vi "host.vi"() -> ()   [LabVIEW 2020]
uses:
  <vilib>/Analysis/baseanly.llb/Real A x B.vi
  <vilib>/Analysis/7linalg.llb/Real Cholesky Factorization.vi
  <vilib>/Analysis/7linalg.llb/Real Transpose Matrix.vi
  <vilib>/Analysis/baseanly.llb/Full Cholesky Factorization.vi
  <vilib>/Analysis/baseanly.llb/Full Real Matrix Cholesky Factorization.vi
  <vilib>/Analysis/baseanly.llb/Real Inverse Matrix.vi
  <vilib>/Analysis/Matrix/Numeric/Conversions/Matrix To Array - RM.vi
  <vilib>/FPGAPlugInAG/cRIO-9035/niLvFpga_Open_cRIO-9035.vi
  <vilib>/rvi/interface/common/dynamic/niFpgaDynamicAddResources.vi
  <vilib>/Utility/error.llb/Error Cluster From Error Code.vi
  <vilib>/rvi/errors/niLvFpgaAdjustHostInterfaceError.vi
  <vilib>/FPGAPlugInAG/Dynamic/niLvFpga_Run_Dynamic.vi
  <vilib>/FPGAPlugInAG/Dynamic/niLvFpga_Close_Dynamic.vi
  <vilib>/rvi/interface/nirviOpenFPGA/nirviOpenFPGA.xnode
  FPGA Bitfiles/labviewfpgacheck_FPGATarget_target_WT8zXaMNSug.lvbitx
  target.vi
  <vilib>/rvi/interface/nirviMethod/nirviMethod.xnode
  <vilib>/rvi/interface/nirviCloseFPGA/nirviCloseFPGA.xnode
  <vilib>/FPGAPlugInAG/Dynamic/niLvFpga_WriteFifo_Dynamic.vi
  <vilib>/rvi/errors/niLvFpgaMergeErrorWithErrorCode.vi
  <vilib>/FPGAPlugInAG/Dynamic/niLvFpga_ReadFifo_Dynamic.vi
  <vilib>/Analysis/NI_AALBase.lvlib
  <vilib>/Analysis/NI_AALPro.lvlib
  <vilib>/Analysis/Matrix/NI_Matrix.lvlib
panel:
  out "B - LabVIEW code":dbl[][](array[numeric])
  out "sum of error":dbl
  out "B - FPGA code":sgl[][](array[numeric])
  out "A":sgl[][](array[numeric])
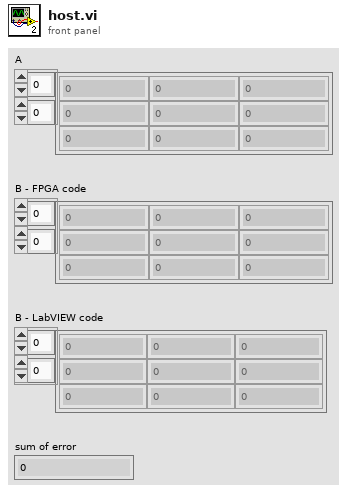
[diagram p1: front panel]
types:
  T1 = typedef "NI_Matrix.lvlib/RealMatrix.ctl" = dbl[][]
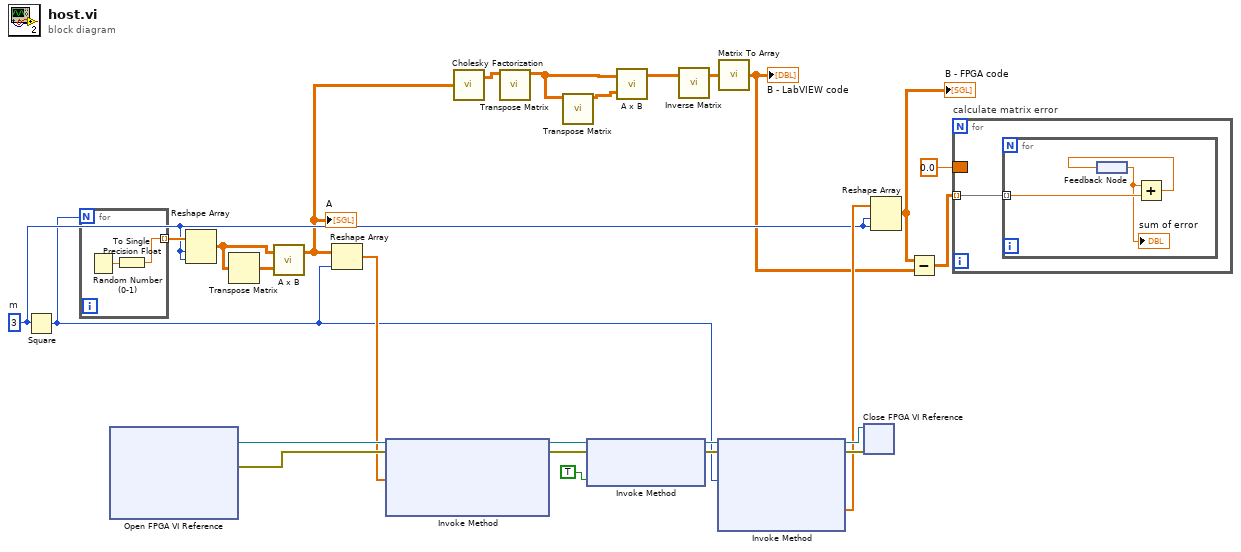
[diagram p0: block diagram]
diagram:
  w10 = 3  # m
  n1 = Square(x=w10) -> (x^2=w9:i32)
  n2 = for {
    N: w9 -> [_]
    tunnel: [w27] -> w13 mode=indexing
    n3 = Random Number (0-1)() -> (number: 0 to 1=w28:dbl)
    n4 = To Single Precision Float(number=w28) -> (single precision float=w27:sgl)
  }
  n5 = xnode "Open FPGA VI Reference"() -> ("FPGA VI Reference Out"=w25:refnum<k20>, "error out"=w24:errorcluster)  [unwired: 2 in]
  n6 = Reshape Array(w13, w10, w10) -> (w11:sgl[][])
  n7 = Transpose Matrix(1:w11) -> (0:w12:dbl[][])
  n8 = call-poly <vilib>:"A x B.vi"("B"=w12, "A"=w11) -> ("A x B"=w6:T1)  [unwired: 1 out]
  "A" <- w6
  n9 = Reshape Array(w6, w9) -> (w19:dbl[])
  n10 = xnode "Invoke Method"("FPGA VI Reference In"=w25, "error in"=w24, "Data"=w19) -> ("FPGA VI Reference Out"=w15:refnum<k20>, "error out"=w14:errorcluster)  [unwired: 1 in, 1 out]
  n11 = call-poly <vilib>:"Cholesky Factorization.vi"("A"=w6) -> ("Cholesky"=w8:T1)  [unwired: 1 out]
  n12 = call-poly <vilib>:"Transpose Matrix.vi"("Input Matrix"=w8) -> ("Matrix Transpose"=w5:T1)  [unwired: 9 in, 1 out]
  n13 = call-poly <vilib>:"Transpose Matrix.vi"("Input Matrix"=w5) -> ("Matrix Transpose"=w7:T1)  [unwired: 9 in, 1 out]
  n14 = xnode "Invoke Method"("FPGA VI Reference In"=w15, "error in"=w14, "Wait Until Done (F)"=TRUE) -> ("FPGA VI Reference Out"=w23:refnum<k20>, "error out"=w22:errorcluster)
  n15 = call-poly <vilib>:"A x B.vi"("B"=w7, "A"=w5) -> ("A x B"=w4:T1)  [unwired: 1 out]
  n16 = call-poly <vilib>:"Inverse Matrix.vi"("Input Matrix"=w4) -> ("Inverse Matrix"=w3:T1)  [unwired: 1 in, 1 out]
  n17 = xnode "Invoke Method"("FPGA VI Reference In"=w23, "error in"=w22, "Number of Elements"=w9) -> ("FPGA VI Reference Out"=w21:refnum<k20>, "error out"=w20:errorcluster, "Data"=w16:sgl[])  [unwired: 1 in, 1 out]
  n18 = call-poly <vilib>:"Matrix To Array.vi"("Real Matrix"=w3) -> ("Real 2D Array"=w2:dbl[][])
  "B - LabVIEW code" <- w2
  n19 = xnode "Close FPGA VI Reference"("FPGA VI Reference In"=w21, "error in"=w20) -> ()  [unwired: 1 out]
  n20 = Reshape Array(w16, w10, w10) -> (w18:sgl[][])
  "B - FPGA code" <- w18
  n21 = Subtract ("Subtract.vi")(x=w18, y=w2) -> (x-y=w17:dbl[][])
  n22 = for "calculate matrix error" {
    tunnel: w17 -> [w29] mode=indexing
    border: 0.0 -> [_]
    n23 = for {
      tunnel: w29 -> [w32] mode=indexing
      n24 = feedback #1() -> (w30:dbl)
      "sum of error" <- w30
      n25 = Add(x=w30, y=w32) -> (x+y=w31:dbl)
      n26 = feedback-in #1(w31) -> ()
    }
  }
